vi "OC2 Setup Output drive.vi"(2 "error in (no error)":errorcluster, 3 "control output values":cluster{"Control  Output":u16, "Output %":dbl} {"Control  Output" items=["Off", "On"]}, 4 "write control output":bool, 5 "VISA resource name":refnum<visa-resource-name>="ASRL1::INSTR") -> (0 "error out":errorcluster, 1 "dup VISA resource name":refnum<visa-resource-name>)   [LabVIEW 2009]
doc: "TCM Setup Output drivel.vi\n\nVI that sets the output drive information, accepts a cluster that contains the following variables:\ncontrol output - sets the output control to on, controls the tcm as per the settings in contol type vi\noutput % - will set the output to the percentage entered when control outputis off\n\nCOPYRIGHT ELECTRON DYNAMICS LTD"
panel:
  out "write data":string
  # "Set output drive variables"
  # "V1.02"
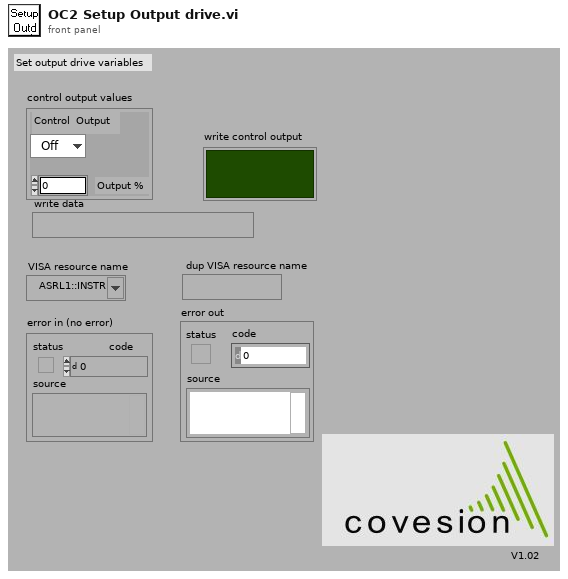
[diagram p1: front panel]
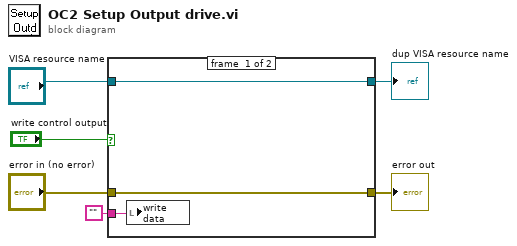
[diagram p0: block diagram]
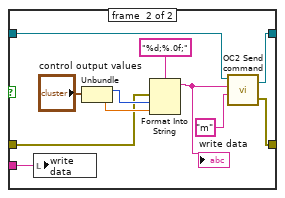
[diagram p2: hidden frame]
diagram:
  n1 = case shown="True" "write control output" {
    tunnel: "error in (no error)" -> [w8 w14]
    tunnel: "VISA resource name" -> [w9 w13]
    tunnel: [w9 w12] -> w4
    tunnel: [w8 w11] -> w3
    tunnel: "" -> [w7 w10]
    frame #0 {
      n2 = local write "write data"(w7) -> ()
    }
    frame #1 {
      n3 = local write "write data"(w10) -> ()
      n4 = Unbundle("control output values") -> ("Control  Output"=w16:u16, "Output %"=w15:dbl)
      n5 = Format Into String(format string="%d;%.0f;", error in=w14, w16, w15) -> (resulting string=w18:string)  [unwired: 1 in, 1 out]
      "write data" <- w18
      n6 = call "OC2 Send command.vi"("VISA resource name"=w13, "Command data"=w18, "Command"="m") -> ("dup VISA resource name"=w12:refnum<visa-resource-name>, "error out"=w11:errorcluster)  [unwired: 2 in]
    }
  }
  "dup VISA resource name" <- w4
  "error out" <- w3
